vi "Lab6.vi"() -> ()   [LabVIEW 2011]
panel:
  in  "stop":bool
  out "dispersia":dbl format="%#.4g"
  out "suma valorilor":dbl
  out "media":dbl format="%#.4g"
  out "numar de valori":dbl
  out "valoare instatanee":dbl(graph)
  in  "baza":dbl(slide)=4.0458015267175576 scale=0.0..10.0
  out "Numeric":dbl format="%#.4g"
  # "ALEXANDRESCU Anda Cristiana\n334 AB"
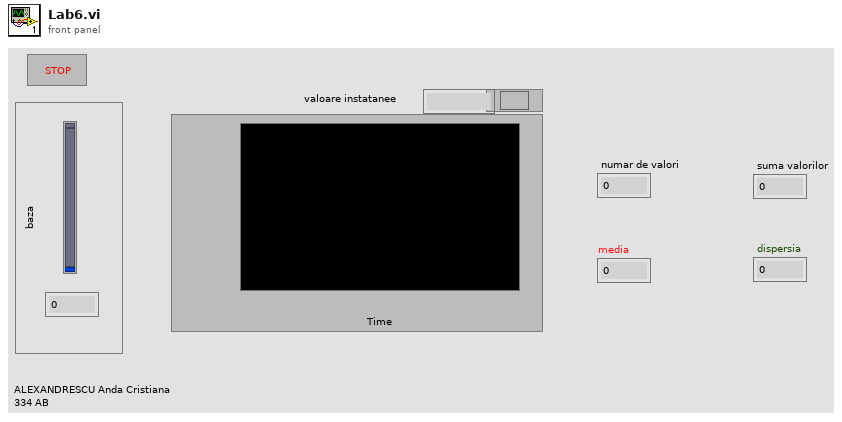
[diagram p1: front panel]
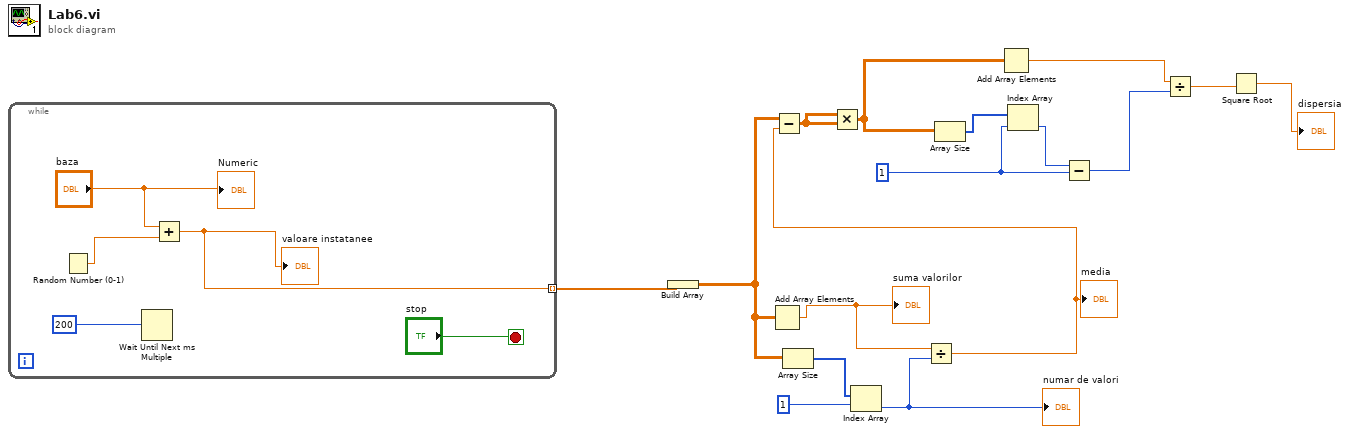
[diagram p0: block diagram]
diagram:
  w10 = 1
  n1 = while {
    tunnel: [w17] -> w16 mode=indexing
    stop <- "stop" stop-if-true
    n2 = Random Number (0-1)() -> (number: 0 to 1=w18:dbl)
    n3 = Wait Until Next ms Multiple(millisecond multiple=200) -> ()  [unwired: 1 out]
    n4 = Add(x="baza", y=w18) -> (x+y=w17:dbl)
    "valoare instatanee" <- w17
    "Numeric" <- "baza"
  }
  n5 = Build Array(w16) -> (w5:dbl[][])
  n6 = Add Array Elements(numeric array=w5) -> (sum=w6:dbl)
  "suma valorilor" <- w6
  n7 = Array Size(array=w5) -> (size(s)=w4:i32[])
  n8 = Index Array(array=w4, index=1) -> (element=w3:i32)
  "numar de valori" <- w3
  n9 = Divide(x=w6, y=w3) -> (x/y=w1:dbl)
  "media" <- w1
  n10 = Subtract(x=w5, y=w1) -> (x-y=w15:dbl[][])
  n11 = Multiply(x=w15, y=w15) -> (x*y=w14:dbl[][])
  n12 = Array Size(array=w14) -> (size(s)=w12:i32[])
  n13 = Add Array Elements(numeric array=w14) -> (sum=w13:dbl)
  n14 = Index Array(array=w12, index=w10) -> (element=w11:i32)
  n15 = Subtract(x=w11, y=w10) -> (x-y=w9:i32)
  n16 = Divide(x=w13, y=w9) -> (x/y=w8:dbl)
  n17 = Square Root(x=w8) -> (sqrt(x)=→"dispersia":dbl)
